vi "Lake Shore Cryotronics 340 Write Curve.vi"() -> ()   [LabVIEW 2019]
doc: "This vi was designed to demonstrate typical usage of sub vi's containing the 340 curve functions.\n\nThis vi performs 3 curve functions, write curve header, write curve point, and save curve to flash. A typical way to use this vi would be to first write a curve header, then write multiple curve points until all points are written. Finally, run the vi selecting the save curve to flash function. Curves are not saved in memory until the save curve to flash function."
uses:
  Lake Shore Cryotronics 340.lvlib
panel:
  in  "Units Value (0.00000)":dbl min=-9999.0 max=9999.0 step=1e-05 format="%.5f"
  in  "Write Curve\nPoint (F: Don't Write Point)":bool
  in  "Write Curve\nHeader (F: Don't Write Header)":bool
  in  "Save Curve\nto Flash (T: Save Curve)":bool=TRUE
  in  "Curve Serial Number (\"\")":string
  in  "Curve Name (\"\")":string
  in  "Limit Value (0.000)":dbl min=0.0 max=1500.0 step=0.001 format="%.3f"
  in  "Curve Data Format (0: mV/K)":u16(ring) items=["mV/K", "V/K", "Ohms/K", "Log Ohms/K", "Log Ohms/Log K"]
  in  "Temp\nCoefficient (0: Negative)":u16(ring) items=["Negative", "Positive"]
  in  "VISA resource name":refnum<visa-resource-name>
  out "error out":errorcluster
  in  "error in (no error)":errorcluster
  in  "Temperature Value (0.00000)":dbl min=-9999.0 max=9999.0 step=1e-05 format="%.5f"
  in  "Index (1)":dbl=1.0 min=1.0 max=200.0 step=1.0
  in  "Curve (21)":dbl=21.0 min=21.0 max=60.0 step=1.0
  # "Copyright 2005. National Instruments Corporation"
  # "Save Curve\nDon't Save Curve"
  # "Write Header\nDon't Write Header"
  # "Write Point\nDon't Write Point"
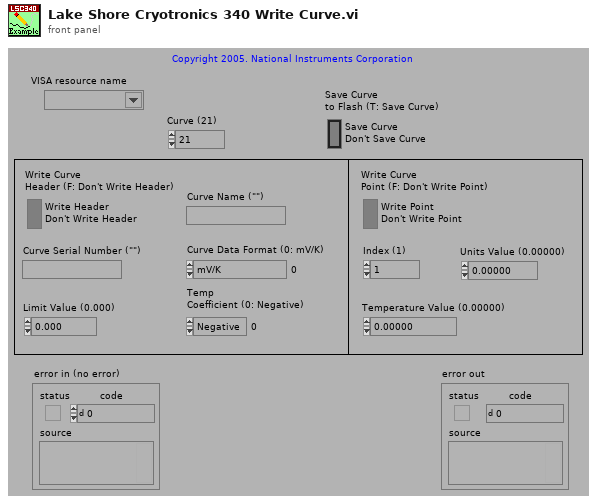
[diagram p1: front panel]
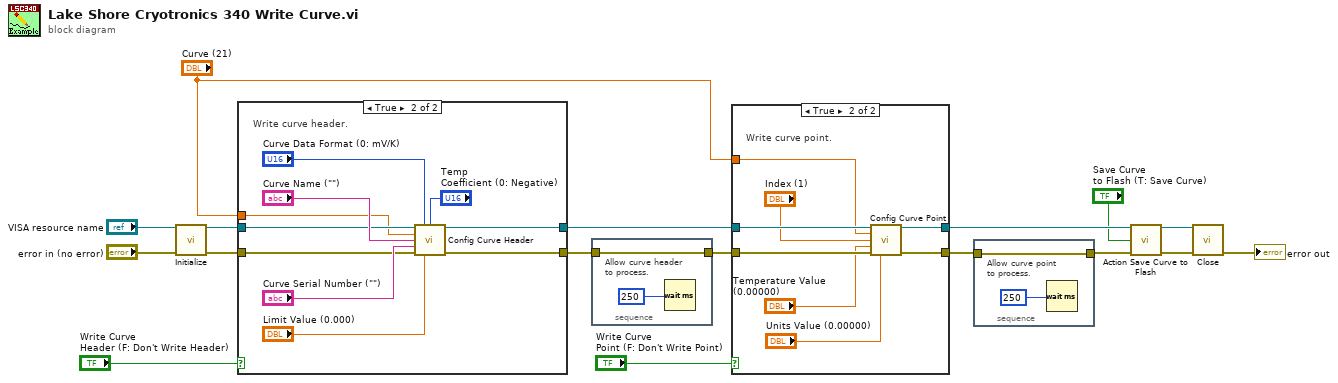
[diagram p0: block diagram]
diagram:
  n1 = call "Initialize.vi"("VISA resource name"="VISA resource name", "error in (no error)"="error in (no error)") -> ("VISA resource name out"=w4:refnum<visa-resource-name>, "error out"=w5:errorcluster)  [unwired: 12 in]
  n2 = case shown="True" "Write Curve\nHeader (F: Don't Write Header)" {
    tunnel: w4 -> [w19 w24]
    tunnel: w5 -> [w18 w23]
    tunnel: [w19 w22] -> w16
    tunnel: [w18 w21] -> w11
    tunnel: "Curve (21)" -> [_ w20]
    frame False {
      # "Don't write curve header."
    }
    frame True {
      # "Write curve header."
      n3 = call "Config Curve Header.vi"("VISA resource name"=w24, "Curve Data Format (0: mV/K)"="Curve Data Format (0: mV/K)", "Temp Coefficient (0: Negative)"="Temp\nCoefficient (0: Negative)", "Curve (21)"=w20, "Curve Name (\"\")"="Curve Name (\"\")", "Curve Serial Number (\"\")"="Curve Serial Number (\"\")", "error in (no error)"=w23, "Limit Value (0.000)"="Limit Value (0.000)") -> ("VISA resource name out"=w22:refnum<visa-resource-name>, "error out"=w21:errorcluster)  [unwired: 6 in]
    }
  }
  n4 = stacked-sequence {
    tunnel: w11 -> [w30]
    tunnel: [w30] -> w10
    frame #0 {
      # "Allow curve header\nto process."
      n5 = Wait (ms)(milliseconds to wait=u32 250) -> ()  [unwired: 1 out]
    }
  }
  n6 = case shown="True" "Write Curve\nPoint (F: Don't Write Point)" {
    tunnel: w16 -> [w33 w41]
    tunnel: w10 -> [w32 w40]
    tunnel: "Curve (21)" -> [_ w37]
    tunnel: [w33 w36] -> w13
    tunnel: [w32 w35] -> w9
    frame False {
      # "Don't Write curve point."
    }
    frame True {
      # "Write curve point."
      n7 = call "Config Curve Point.vi"("VISA resource name"=w41, "Curve (21)"=w37, "Index (1)"="Index (1)", "Temperature \nValue (0.00000)"="Temperature Value (0.00000)", "error in (no error)"=w40, "Units Value (0.00000)"="Units Value (0.00000)") -> ("VISA resource name out"=w36:refnum<visa-resource-name>, "error out"=w35:errorcluster)  [unwired: 8 in]
    }
  }
  n8 = stacked-sequence {
    tunnel: w9 -> [w42]
    tunnel: [w42] -> w8
    frame #0 {
      # "Allow curve point\nto process."
      n9 = Wait (ms)(milliseconds to wait=u32 250) -> ()  [unwired: 1 out]
    }
  }
  n10 = call "Action Save Curve to Flash.vi"("VISA resource name"=w13, "Save Curve to Flash (T: Save)"="Save Curve\nto Flash (T: Save Curve)", "error in (no error)"=w8) -> ("VISA resource name out"=w3:refnum<visa-resource-name>, "error out"=w2:errorcluster)  [unwired: 11 in]
  n11 = call "Close.vi"("VISA resource name"=w3, "error in (no error)"=w2) -> ("error out"=→"error out":errorcluster)  [unwired: 13 in]
